vi "Exercise 3.2 – MathScript.vi"() -> ()   [LabVIEW 2024]
panel:
  out "Frequency":dbl
  out "Amplitude":dbl
  in  "Frequency In":dbl(knob)=20.373516313769578 scale=0.0..100.0
  out "Waveform Graph":dynamicdata(graph)
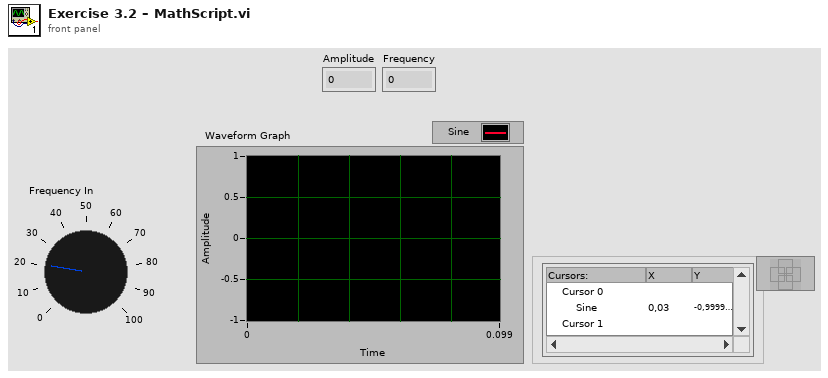
[diagram p1: front panel]
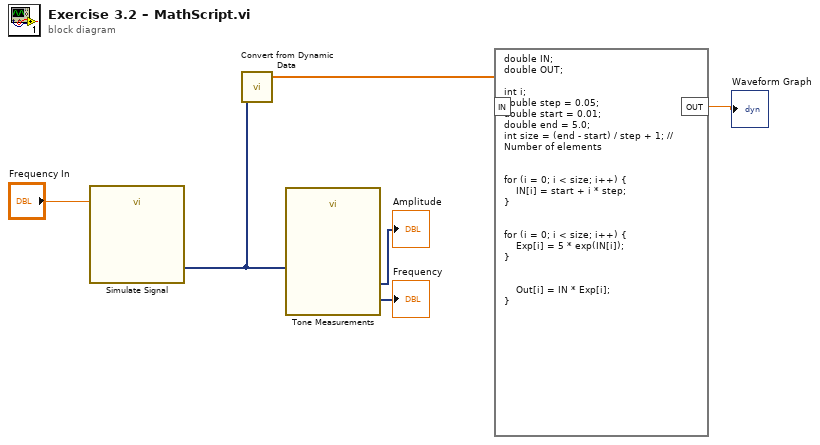
[diagram p0: block diagram]
diagram:
  n1 = call "Simulate Signal"("Frequency"="Frequency In") -> ("Sine"=w3:dynamicdata)  [unwired: 13 in, 1 out]
  n2 = call "Convert from Dynamic Data"("Dynamic Data Type"=w3) -> ("Array"=w2:dbl[])  [unwired: 3 in]
  n3 = call "Tone Measurements"("Signals"=w3) -> ("Frequency"=→"Frequency":dynamicdata, "Amplitude"=→"Amplitude":dynamicdata)  [unwired: 8 in, 1 out]
  n4 = formula code="double IN;\ndouble OUT;\n\nint i;\ndouble step = 0.05;\ndouble start = 0.01;\ndouble end = 5.0;\nint size = (end - start) / step + 1; // Number of elements\n\n\nfor (i = 0; i < size; i++) {\n    IN[i] = start + i * step;\n}\n\n\nfor (i = 0; i < size; i++) {\n    Exp[i] = 5 * exp(IN[i]);\n}\n\n\n    Out[i] = IN * Exp[i];\n}"("IN"=w2) -> ("OUT"=→"Waveform Graph":dbl)
